vi "CreateControlFromReference.vi"(3 "error in (no error)":errorcluster, 4 "Src CtlRef":refnum<vi>, 5 "VI Refnum":refnum<vi>) -> (0 "error out":errorcluster, 1 "New Object Ref":refnum<vi>, 2 "VI Refnum out":refnum<vi>)   [LabVIEW 2021, in "MemberVICreation.lvlib" / "BaseAccessorScripter.lvclass"]
uses:
  <resource>/Framework/Providers/LVClassLibrary/NewAccessors/BaseAccessorScripter/BaseAccessorScripter.lvclass
  <vilib>/Utility/miscctls.llb/LVPointTypeDef.ctl
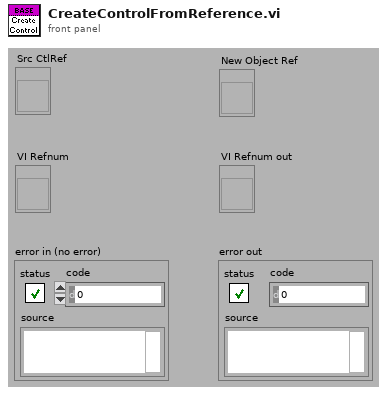
[diagram p1: front panel]
types:
  T1 = typedef "LVPointTypeDef.ctl" = cluster{"Horizontal":i16, "Vertical":i16}
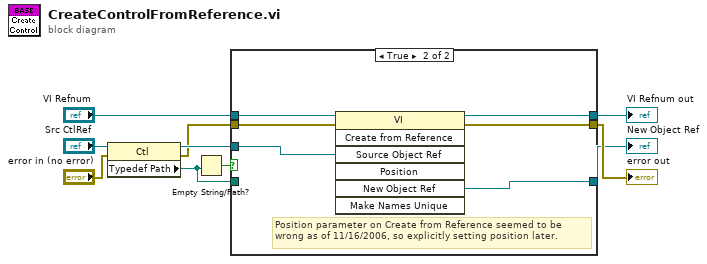
[diagram p0: block diagram]
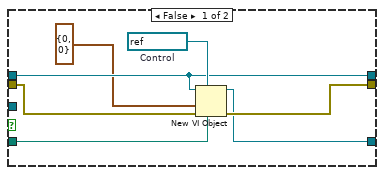
[diagram p2: hidden frame]
diagram:
  n1 = property class="Ctl"(reference="Src CtlRef", error in="error in (no error)") -> (reference out=w4:refnum<vi>, error out=w3:errorcluster, "Typedef Path"=w1:path)
  n2 = Empty String/Path?(string/path=w1) -> (empty?=w2:bool)
  n3 = case shown="True" w2 {
    tunnel: [w12 w23] -> w10
    tunnel: [w14 w22] -> w9
    tunnel: [w13 w21] -> w8
    tunnel: "VI Refnum" -> [w12 w20]
    tunnel: w4 -> [_ w19]
    tunnel: w3 -> [w15 w18]
    tunnel: w1 -> [w16 _]
    frame False {
      w17 = refnum<vi> refnum  # Control
      n4 = New VI Object(vi object class=w17, owner refnum=w12, position/next to=T1 {"Horizontal"=0, "Vertical"=0} ("relative position/next to refnum"), 6:w16, 8:w15) -> (object refnum=w13:refnum<vi>, 0:w14:errorcluster)  [unwired: 3 out]
    }
    frame True {
      # "Position parameter on Create from Reference seemed to be \nwrong as of 11/16/2006, so explicitly setting position later."
      n5 = invoke class="VI" method="Create from Reference"(reference=w20, error in=w18, "Source Object Ref"=w19) -> (reference out=w23:refnum<vi>, error out=w22:errorcluster, "New Object Ref"=w21:refnum<vi>)  [unwired: 4 in, 4 out]
    }
  }
  "VI Refnum out" <- w10
  "error out" <- w9
  "New Object Ref" <- w8
